vi "Digital Format String.vi"(7 "Representation":T1, 10 "Format String in":string) -> (1 "Force Radix Visible":bool, 2 "Format String out":string)   [LabVIEW 2019, in "Quick Format QD.lvlib"]
doc: "Converts the Format String input into a Format String a digital control or constant can accept."
uses:
  Quick Format QD.lvlib
  <vilib>/numeric/LVNumericRepresentation.ctl
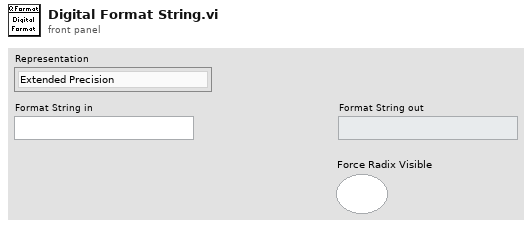
[diagram p1: front panel]
types:
  T1 = typedef "LVNumericRepresentation.ctl" = enum32{"Extended Precision", "Double Precision", "Single Precision", "Long", "Word", "Byte", "Unsigned Long", "Unsigned Word", "Unsigned Byte", "Complex Extended", "Complex Double", "Complex Single", "Quad", "Unsigned Quad", "Fixed-Point"}
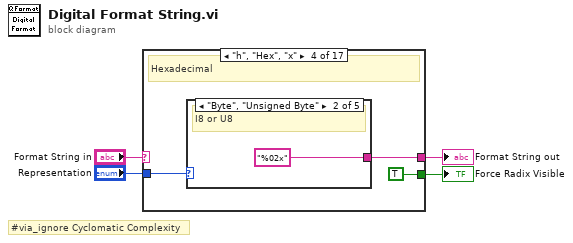
[diagram p0: block diagram]
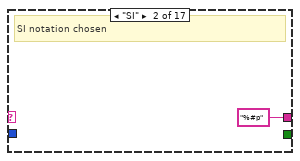
[diagram p3: hidden frame]
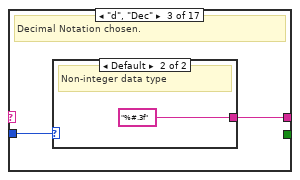
[diagram p4: hidden frame]
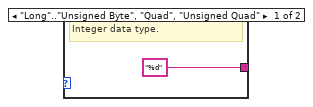
[diagram p5: hidden frame]
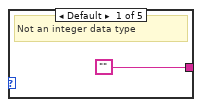
[diagram p6: hidden frame]
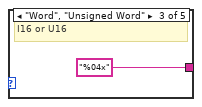
[diagram p7: hidden frame]
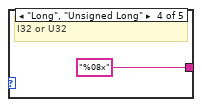
[diagram p8: hidden frame]
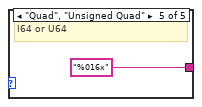
[diagram p9: hidden frame]
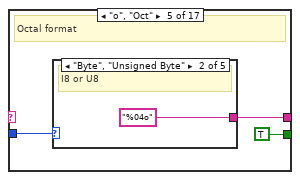
[diagram p10: hidden frame]
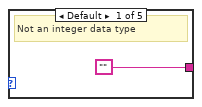
[diagram p11: hidden frame]
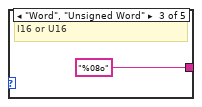
[diagram p12: hidden frame]
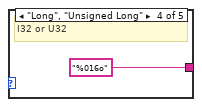
[diagram p13: hidden frame]
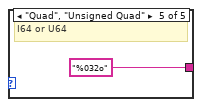
[diagram p14: hidden frame]
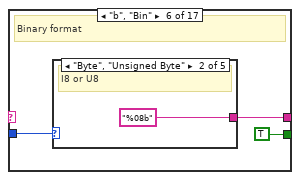
[diagram p15: hidden frame]
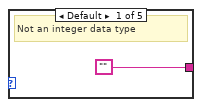
[diagram p16: hidden frame]
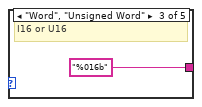
[diagram p17: hidden frame]
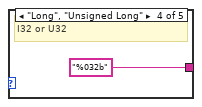
[diagram p18: hidden frame]
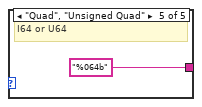
[diagram p19: hidden frame]
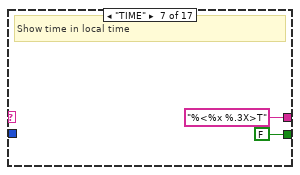
[diagram p20: hidden frame]
diagram:
  # "#via_ignore Cyclomatic Complexity"
  n1 = case shown="\"h\", \"Hex\", \"x\"" "Format String in" {
    selector: "Format String in" -> [w5 _ _ _ _ _ _ _ _ _ _ _ _ _ _ _ _]
    tunnel: "Representation" -> [_ _ w8 w13 w21 w29 _ _ _ _ _ _ _ _ _ _ _]
    tunnel: [w5 "%#p" ("Format String") w7 w12 w20 w28 "%<%x %.3X>T" ("Format String") "%^<%x %.3X %Z>T" ("Format String") "%#pHz" ("Format String") "%#fdB" ("Format String") "%#fdBm" ("Format String") "%#fdBc" ("Format String") "%#ps" ("Format String") "%#pV" ("Format String") "%#pA" ("Format String") "%#pOhm" ("Format String") "%#pW" ("Format String")] -> w2
    tunnel: [_ _ _ TRUE TRUE TRUE FALSE FALSE _ _ _ _ _ _ _ _ _] -> w1
    frame Default {
      # "Custom Format String.  Write FormatString directly."
    }
    frame "SI" {
      # "SI notation chosen"
    }
    frame "d", "Dec" {
      # "Decimal Notation chosen."
      n2 = case shown="Default" w8 {
        tunnel: ["%d" ("Format String") "%#.3f" ("Format String")] -> w7
        frame "Long".."Unsigned Byte", "Quad", "Unsigned Quad" {
          # "Integer data type."
        }
        frame Default {
          # "Non-integer data type"
        }
      }
    }
    frame "h", "Hex", "x" {
      # "Hexadecimal"
      n3 = case shown="\"Byte\", \"Unsigned Byte\"" w13 {
        tunnel: ["" ("Empty String Constant") "%02x" ("Format String") "%04x" ("Format String") "%08x" ("Format String") "%016x" ("Format String")] -> w12
        frame Default {
          # "Not an integer data type"
        }
        frame "Byte", "Unsigned Byte" {
          # "I8 or U8"
        }
        frame "Word", "Unsigned Word" {
          # "I16 or U16"
        }
        frame "Long", "Unsigned Long" {
          # "I32 or U32"
        }
        frame "Quad", "Unsigned Quad" {
          # "I64 or U64"
        }
      }
    }
    frame "o", "Oct" {
      # "Octal format"
      n4 = case shown="\"Byte\", \"Unsigned Byte\"" w21 {
        tunnel: ["" ("Empty String Constant") "%04o" ("Format String") "%08o" ("Format String") "%016o" ("Format String") "%032o" ("Format String")] -> w20
        frame Default {
          # "Not an integer data type"
        }
        frame "Byte", "Unsigned Byte" {
          # "I8 or U8"
        }
        frame "Word", "Unsigned Word" {
          # "I16 or U16"
        }
        frame "Long", "Unsigned Long" {
          # "I32 or U32"
        }
        frame "Quad", "Unsigned Quad" {
          # "I64 or U64"
        }
      }
    }
    frame "b", "Bin" {
      # "Binary format"
      n5 = case shown="\"Byte\", \"Unsigned Byte\"" w29 {
        tunnel: ["" ("Empty String Constant") "%08b" ("Format String") "%016b" ("Format String") "%032b" ("Format String") "%064b" ("Format String")] -> w28
        frame Default {
          # "Not an integer data type"
        }
        frame "Byte", "Unsigned Byte" {
          # "I8 or U8"
        }
        frame "Word", "Unsigned Word" {
          # "I16 or U16"
        }
        frame "Long", "Unsigned Long" {
          # "I32 or U32"
        }
        frame "Quad", "Unsigned Quad" {
          # "I64 or U64"
        }
      }
    }
    frame "TIME" {
      # "Show time in local time"
    }
    frame "UTC" {
      # "Show time in UTC"
    }
    frame "freq" {
      # "Frequency value.  Show Hz units."
    }
    frame "db" {
      # "RF power value.  Show dB units."
    }
    frame "dbm" {
      # "RF power relative to 1mW.  Show dBm units."
    }
    frame "dbc" {
      # "RF power relative to carrier.  Show dBc units."
    }
    frame "sec" {
      # "Time value.  Show seconds units."
    }
    frame "volt" {
      # "Voltage value.  Show Volt units."
    }
    frame "amp" {
      # "Current value.  Show Amp units."
    }
    frame "ohm" {
      # "Resistance value.  Show Ohm units."
    }
    frame "watt" {
      # "Power value.  Show Watt units."
    }
  }
  "Format String out" <- w2
  "Force Radix Visible" <- w1
